vi "Set Discover Channels.vi"(8 "error in (no error)":errorcluster, 10 "discover channels":bool, 11 "references in":T1) -> (0 "error out":errorcluster, 3 "references out":T1)   [LabVIEW 2013, in "Scan Engine configuration.lvclass"]
uses:
  Scan Engine configuration.lvclass
  <vilib>/NI/DCAF/Tag Editor Core/Table API/Table Manager/object ref.ctl
  <vilib>/NI/DCAF/Tag Editor Core/Configuration Editor/Classes/Engine Parent/Engine Parent Editor Node.lvclass
  <vilib>/NI/DCAF/Tag Editor Core/Configuration Editor/Classes/Module editor node/module editor node.lvclass
  <vilib>/NI/DCAF/Tag Editor Core/Configuration Editor/Classes/Module editor node/Read Module Configuration.vi
  <vilib>/NI/DCAF/Tag Editor Core/Configuration Editor/Classes/Module editor node/Write Module Configuration.vi
  <vilib>/NI/Tag Bus Module Framework/module configuration/TBM module configuration.lvclass
  <vilib>/NI/DCAF/Tag Editor Core/Table API/Table Manager/Table Manager.lvclass
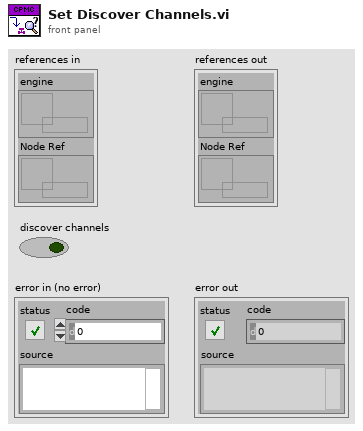
[diagram p1: front panel]
types:
  T1 = typedef "Table Manager.lvlib/Table Manager.lvclass/object ref.ctl" = cluster{"engine":refnum<data-value>, "Node Ref":refnum<data-value>}
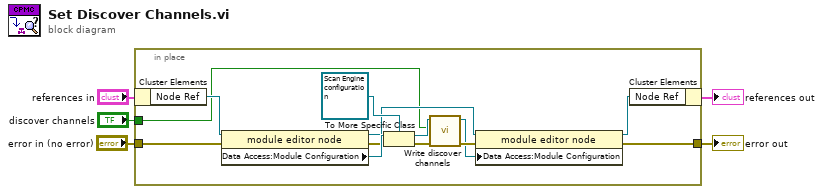
[diagram p0: block diagram]
diagram:
  n1 = in-place {
    in-place-border: "error in (no error)" -> [w13]
    in-place-border: [w11] -> w3
    in-place-border: "discover channels" -> [w6]
    n2 = in-place-cluster #1("references in") -> ("Node Ref"=w17:refnum<data-value>)
    n3 = property class="module editor node"(reference=w17, error in=w13) -> (reference out=w15:refnum<data-value>, error out=w12:errorcluster, "Data Access:Module Configuration"=w16:refnum<class "TBM module configuration.lvclass">)
    n4 = To More Specific Class(target class=refnum<class "Scan Engine configuration.lvclass"> refnum ("Scan Engine configuration"), reference=w16, error in=w12) -> (specific class reference=w10:refnum<class "Scan Engine configuration.lvclass">, error out=w9:errorcluster)
    n5 = call-dynamic "Write discover channels.vi"("error in (no error)"=w9, "discover channels"=w6, "Scan Engine configuration1 in"=w10) -> ("error out"=w8:errorcluster, "Scan Engine configuration1 out"=w7:refnum<class "Scan Engine configuration.lvclass">)  [unwired: 7 in]
    n6 = property class="module editor node"(reference=w15, error in=w8, "Data Access:Module Configuration"=w7) -> (reference out=w14:refnum<data-value>, error out=w11:errorcluster)
    n7 = in-place-cluster #1("Node Ref"=w14) -> (→"references out":T1)
  }
  "error out" <- w3
